vi "get_specified_KeyParams_from_GFG.vi"(7 "Fetch Source (Default:GFGCore)":enum16{"GFG Core", "GFG Translator"}(ring), 11 "Key Parameter Type":string) -> (3 "Requested Key Parameters OUT":cluster{T1[], string})   [LabVIEW 2012]
uses:
  Custom Controls and Typedefs/Calibration Key Param structure.ctl
  <vilib>/Utility/VariantDataType/Type.ctl
  Custom Controls and Typedefs/Galvo (Stim Path) Key Parameters.ctl
  Custom Controls and Typedefs/Galvo Key Parameters.ctl
  Custom Controls and Typedefs/Reso Key Parameters.ctl
  GFG/GFG Translator Wrapper/GFGTranslator_Action.ctl
  GFG/GFG Translator Wrapper/GFGTranslator_Datatype.ctl
  <vilib>/Utility/VariantDataType/VariantType.lvlib
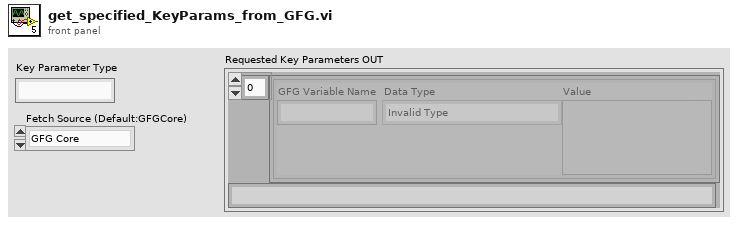
[diagram p1: front panel]
types:
  T1 = typedef "Calibration Key Param structure.ctl" = cluster{"GFG Variable Name":string, "Data Type":T2, "Value":variant}
  T2 = typedef "VariantType.lvlib/Type.ctl" = enum8{"Invalid Type", "Void", "I8", "I16", "I32", "I64", "U8", "U16", "U32", "U64", "Single Float", "Double Float", "Extended Float", "Single Complex", "Double Complex", "Extended Complex", "Enum U8", "Enum U16", "Enum U32", "Enum U64", "Single Float With Unit", "Double Float With Unit", "Extended Float With Unit", "Single Complex with Unit", "Double Complex with Unit", "Extended Complex with Unit", "Boolean", "String", "Path", "Picture", "Tag", "Array", "Cluster", "Variant", "LV Variant", "Waveform", "Timestamp", "Digital Waveform", "Digital Data", "ExpressData", "Refnum", "External Data", "VI", "Poly VI", "LabVIEW Class Instance", "Fixed Point"}
  T3 = typedef "Reso Key Parameters.ctl" = T1[]
  T4 = typedef "Galvo Key Parameters.ctl" = T1[]
  T5 = typedef "Galvo (Stim Path) Key Parameters.ctl" = T1[]
  T6 = typedef "GFGTranslator_Datatype.ctl" = enum16{"String", "Path (String)", "Numeric", "Boolean", "Set_BoolRef (use boolean data)", "Get_Variant", "Get_2DArray (I16)", "Get_Image_2DArray (I16)", "Get_Version (String)", "Get_All GFG variables (String)"}
  T7 = typedef "GFGTranslator_Action.ctl" = enum16{"Get", "Set"}
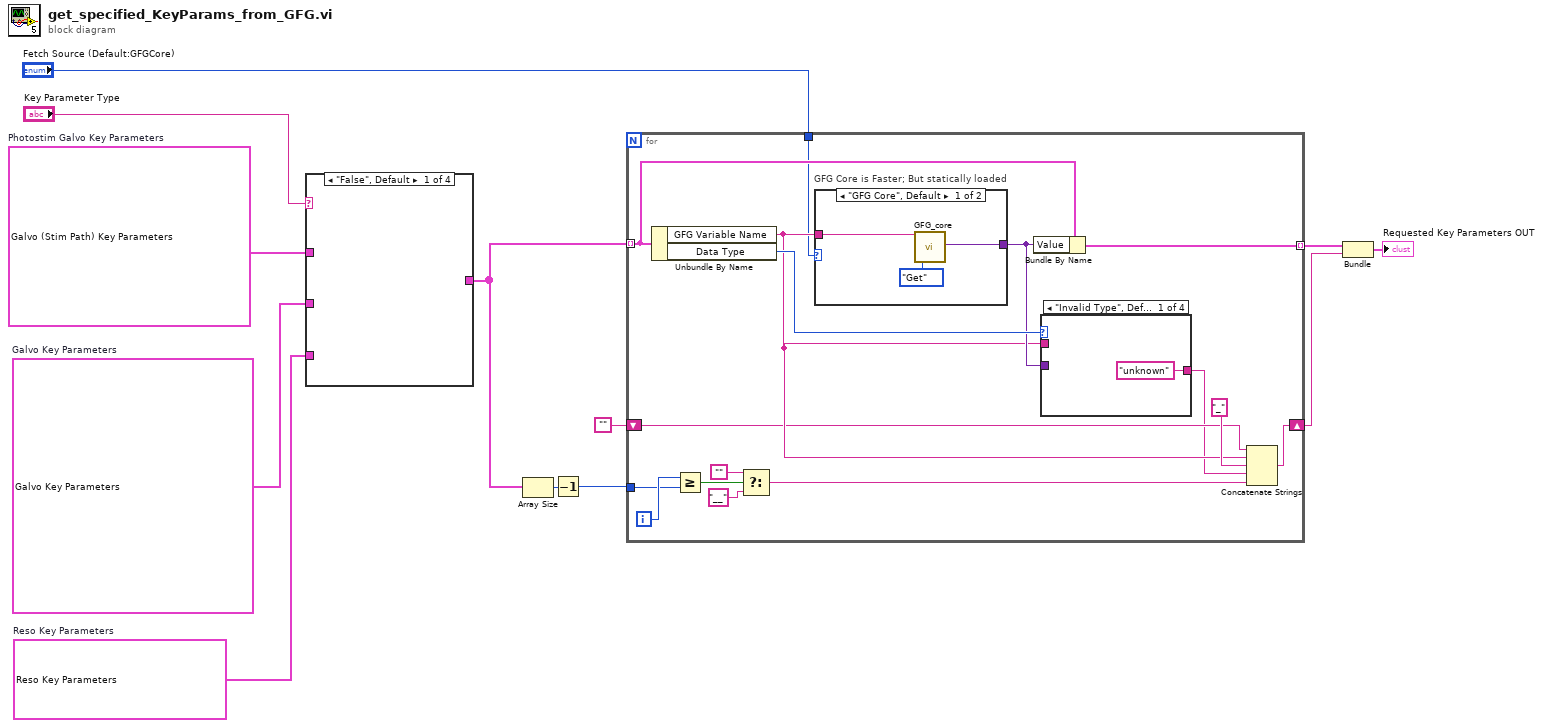
[diagram p0: block diagram]
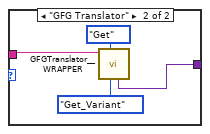
[diagram p2: hidden frame]
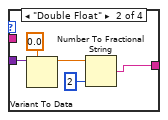
[diagram p3: hidden frame]
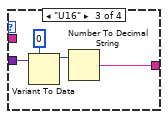
[diagram p4: hidden frame]
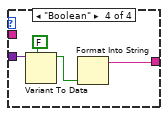
[diagram p5: hidden frame]
diagram:
  w9 = T3 [{"GFG Variable Name"="x.voltage", "Data Type"=enum."Double Float", "Value"=variant}, {"GFG Variable Name"="y.voltage", "Data Type"=enum."Double Float", "Value"=variant}, {"GFG Variable Name"="x.correction", "Data Type"=enum."Double Float", "Value"=variant}]  # Reso Key Parameters
  w10 = T4 [{"GFG Variable Name"="x.voltage", "Data Type"=enum."Double Float", "Value"=variant}, {"GFG Variable Name"="y.voltage", "Data Type"=enum."Double Float", "Value"=variant}, {"GFG Variable Name"="x.volt.offset", "Data Type"=enum."Double Float", "Value"=variant}, {"GFG Variable Name"="y.volt.offset", "Data Type"=enum."Double Float", "Value"=variant}, {"GFG Variable Name"="speed.mode", "Data Type"=enum."U16", "Value"=variant}, {"GFG Variable Name"="fill.fraction", "Data Type"=enum."Double Float", "Value"=variant}, {"GFG Variable Name"="x.bidirectional", "Data Type"=enum."Boolean", "Value"=variant}, {"GFG Variable Name"="y.bidirectional", "Data Type"=enum."Boolean", "Value"=variant}, {"GFG Variable Name"="x.invert.image", "Data Type"=enum."Boolean", "Value"=variant}, {"GFG Variable Name"="y.invert.image", "Data Type"=enum."Boolean", "Value"=variant}]  # Galvo Key Parameters
  w11 = T5 [{"GFG Variable Name"="x.voltage", "Data Type"=enum."Double Float", "Value"=variant}, {"GFG Variable Name"="y.voltage", "Data Type"=enum."Double Float", "Value"=variant}, {"GFG Variable Name"="x.volt.offset", "Data Type"=enum."Double Float", "Value"=variant}, {"GFG Variable Name"="y.volt.offset", "Data Type"=enum."Double Float", "Value"=variant}, {"GFG Variable Name"="fill.fraction", "Data Type"=enum."Double Float", "Value"=variant}, {"GFG Variable Name"="x.invert.image", "Data Type"=enum."Boolean", "Value"=variant}, {"GFG Variable Name"="y.invert.image", "Data Type"=enum."Boolean", "Value"=variant}]  # Photostim Galvo Key Parameters
  n1 = case shown="\"False\", Default" "Key Parameter Type" {
    tunnel: w11 -> [_ w13 _ _]
    tunnel: w10 -> [_ _ w14 _]
    tunnel: w9 -> [_ _ _ w15]
    tunnel: [_ w13 w14 w15] -> w6
    frame "False", Default {
    }
    frame "Stimulation Path Galvo" {
    }
    frame "Imaging Path Galvo" {
    }
    frame "Imaging Path Reso" {
    }
  }
  n2 = Array Size(array=w6) -> (size(s)=w7:i32)
  n3 = Decrement(x=w7) -> (x-1=w5:i32)
  n4 = for {
    tunnel: w6 -> [w31] mode=indexing
    tunnel: [w30] -> w4 mode=indexing
    shift-right: [w17] -> w3
    shift-left: "" -> [w20]
    tunnel: w5 -> [w25]
    tunnel: "Fetch Source (Default:GFGCore)" -> [w16]
    i -> [w26]
    n5 = Unbundle By Name(w31) -> ("GFG Variable Name"=w21:string, "Data Type"=w24:T2)
    n6 = Greater Or Equal?(x=w26, y=w25) -> (x >= y?=w29:bool)
    n7 = Select(t="", s=w29, f="__" ("t")) -> (s? t:f=w18:string)
    n8 = case "GFG Core is Faster; But statically loaded" shown="\"GFG Core\", Default" w16 {
      tunnel: [w33 w35] -> w23
      tunnel: w21 -> [w32 w36]
      frame "GFG Core", Default {
        n9 = call "GFG_core.vi"("Variable Name in"=w32, "Action"=enum16{"Init", "Set", "Get", "Clear"}."Get") -> ("Variant Out"=w33:variant)  [unwired: 11 in, 6 out]
      }
      frame "GFG Translator" {
        n10 = call "GFGTranslator__WRAPPER.vi"("GFGTranslator Datatype"=GFGTranslator_Datatype."Get_Variant", "GFG Translator Action"=GFGTranslator_Action."Get", "GFG Variable Name"=w36) -> ("Variant_Output"=w35:variant)  [unwired: 3 in, 5 out]
      }
    }
    n11 = Bundle By Name(cluster=w31, "Value"=w23) -> (w30:T1)
    n12 = case shown="\"Invalid Type\", Default" w24 {
      tunnel: w21 -> [_ _ _ _]
      tunnel: w23 -> [_ w43 w48 w51]
      tunnel: ["unknown" w40 w45 w49] -> w19
      frame "Invalid Type", Default {
      }
      frame "Double Float" {
        n13 = Variant To Data(type=0.0 ("number"), Variant=w43) -> (data=w41:dbl)  [unwired: 1 in, 1 out]
        n14 = Number To Fractional String(number=w41, precision (6)=i16 2) -> (F-format string=w40:string)  [unwired: 2 in]
      }
      frame "U16" {
        n15 = Variant To Data(type=u16 0 ("number"), Variant=w48) -> (data=w47:u16)  [unwired: 1 in, 1 out]
        n16 = Number To Decimal String(number=w47) -> (decimal integer string=w45:string)  [unwired: 1 in]
      }
      frame "Boolean" {
        n17 = Variant To Data(type=FALSE, Variant=w51) -> (data=w50:bool)  [unwired: 1 in, 1 out]
        n18 = Format Into String(w50) -> (resulting string=w49:string)  [unwired: 3 in, 1 out]
      }
    }
    n19 = Concatenate Strings(w20, w21, "_" ("string"), w19, w18) -> (w17:string)
  }
  n20 = Bundle(w4, w3) -> (→"Requested Key Parameters OUT":cluster{T1[], string})  [unwired: 1 in]
